vi "Write BG_level.vi"(8 "error in (no error)":errorcluster, 10 "BG_level":i32=-1, 11 "Detector in":refnum<class "Detector.lvclass">) -> (0 "error out":errorcluster, 3 "Detector out":refnum<class "Detector.lvclass">)   [LabVIEW 2018, in "Detector.lvclass"]
uses:
  Detector.lvclass
  G:/SD/TRANCON/Classes/GeneralFunctionality/GeneralFunctionality.lvclass
  GeneralFunctionality/GeneralFunctionality.lvclass/GeneralFunctionality.ctl
  Detector.lvclass/Detector.ctl
  dependecies/globalVarII.vi
  Config/Config.lvclass
  GeneralFunctionality/GeneralFunctionality.lvclass
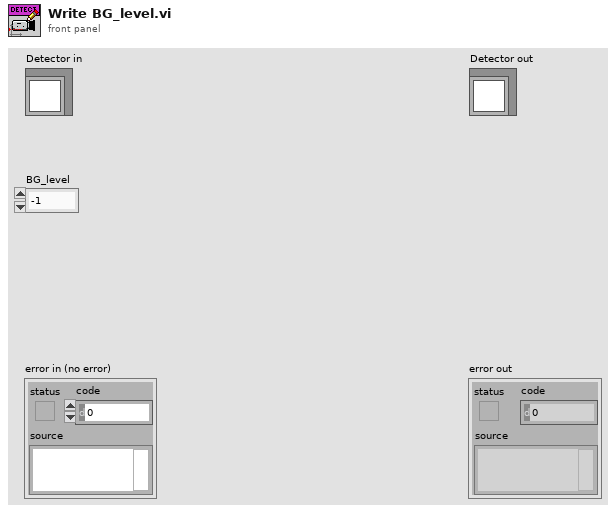
[diagram p1: front panel]
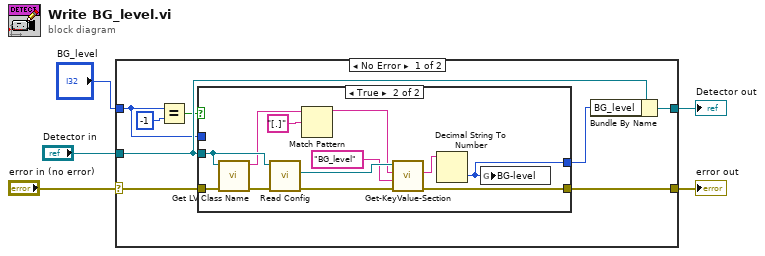
[diagram p0: block diagram]
diagram:
  n1 = case shown="No Error" "error in (no error)" {
    selector: "error in (no error)" -> [w10 w28]
    tunnel: [w12 w28] -> w4
    tunnel: [w13 w29] -> w2
    tunnel: "Detector in" -> [w11 w29]
    tunnel: "BG_level" -> [w6 _]
    frame No Error {
      n2 = Equal?(x=w6, y=-1) -> (x = y?=w7:bool)
      n3 = case shown="True" w7 {
        tunnel: [w14 w25] -> w12
        tunnel: w11 -> [_ w22]
        tunnel: w10 -> [w14 w18]
        tunnel: [w15 w16] -> w9
        tunnel: w6 -> [w15 _]
        frame False {
        }
        frame True {
          n4 = call <vilib>:"Get LV Class Name.vi"("error in (no error)"=w18, "object"=w22) -> ("error out"=w17:errorcluster, "class name"=w21:string)  [unwired: 8 in]
          n5 = call "Read Config.vi"("error in (no error)"=w17, "GeneralFunctionality en entrée"=w22) -> ("error out"=w26:errorcluster, "Config.lvclass"=w27:refnum<class "Config.lvclass">)  [unwired: 7 in, 1 out]
          n6 = Match Pattern(string=w21, regular expression="[.]") -> (before substring=w20:string)  [unwired: 1 in, 3 out]
          n7 = call-dynamic "Get-KeyValue-Section.vi"("error in (no error)"=w26, "Key"="BG_level", "Section"=w20, "Config in"=w27) -> ("error out"=w25:errorcluster, "Value"=w24:string)  [unwired: 5 in, 1 out]
          n8 = Decimal String To Number(string=w24) -> (number=w16:i32)  [unwired: 2 in, 1 out]
          n9 = global write "globalVarII.vi" "BG-level"(w16) -> ()
        }
      }
      n10 = Bundle By Name(cluster=w11, "BG_level"=w9) -> (w13:refnum<class "Detector.lvclass">)
    }
    frame Error {
    }
  }
  "error out" <- w4
  "Detector out" <- w2
